vi "Exercise 4.1 - Creating a SubVI.vi"(10 "y":dbl, 11 "x":dbl) -> (3 "x+y":dbl)   [LabVIEW 2024]
panel:
  out "x+y 3":dbl
  out "x+y 2":dbl
  in  "y 2":dbl
  in  "x 2":dbl
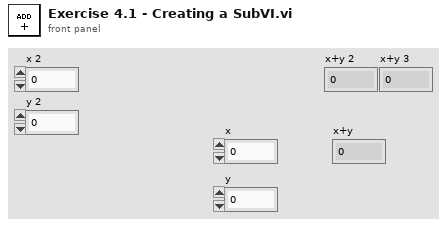
[diagram p1: front panel]
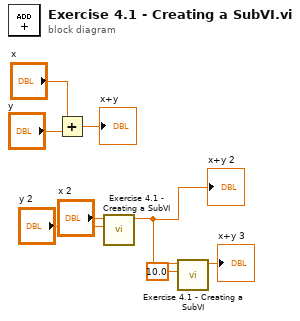
[diagram p0: block diagram]
diagram:
  n1 = Add(x="x", y="y") -> (x+y=→"x+y":dbl)
  n2 = call "Exercise 4.1 - Creating a SubVI.vi"("y"="y 2", "x"="x 2") -> ("x+y"=w2:dbl)  [unwired: 9 in]
  "x+y 2" <- w2
  n3 = call "Exercise 4.1 - Creating a SubVI.vi"("y"=10.0, "x"=w2) -> ("x+y"=→"x+y 3":dbl)  [unwired: 9 in]
